vi "Temperature measurement system - main.vi"() -> ()   [LabVIEW 2022 SP3]
panel:
  in  "Speed":u32=100
  out "Thermometer":dbl(slide) caption="Temperature" scale=0.0..100.0
  out "Tea Ready":bool
  out "Elapsed Time Clock":dbl(knob) caption="Elapsed Time" scale=0.0..28800.0 scale format="%<%H:%M>t"
  out "Elapsed Time (s)":dbl format="%#_3g"
  in  "Device name":tag="myDAQ1"
  in  "B":dbl=3950.0
  in  "R0":dbl=10000.0
  in  "Stop":bool
  in  "Tab Control":enum32{"Voltage", "Resistance", "Temperature"}(tab)
  out "Voltage Chart":dbl(graph)
  out "Resistance Chart":dbl(graph)
  out "Temperature Chart":dbl(graph)
  out "Temperature":dbl format="%#_3g"
  in  "R2":dbl=10000.0
  out "Resistance":dbl
  out "Voltage 1":dbl format="%#_2g"
  out "Voltage 2":dbl format="%#_2g"
  # "Configuration"
  # "Results"
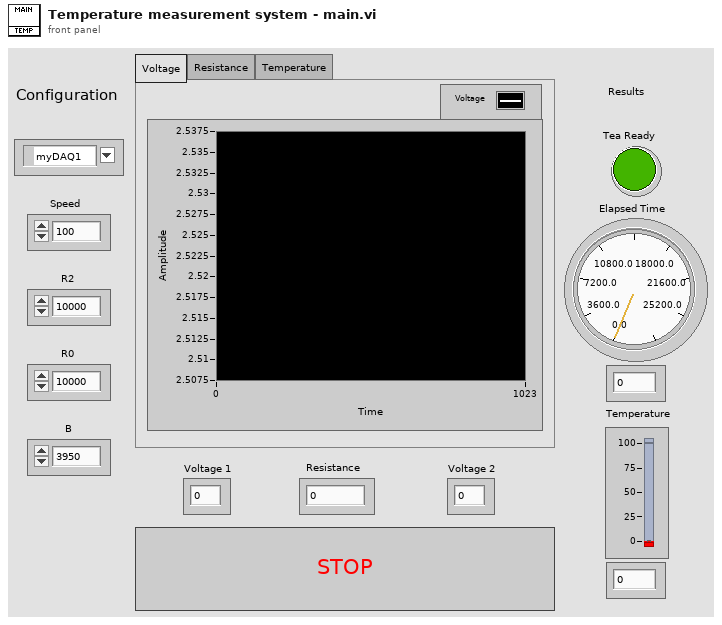
[diagram p1: front panel]
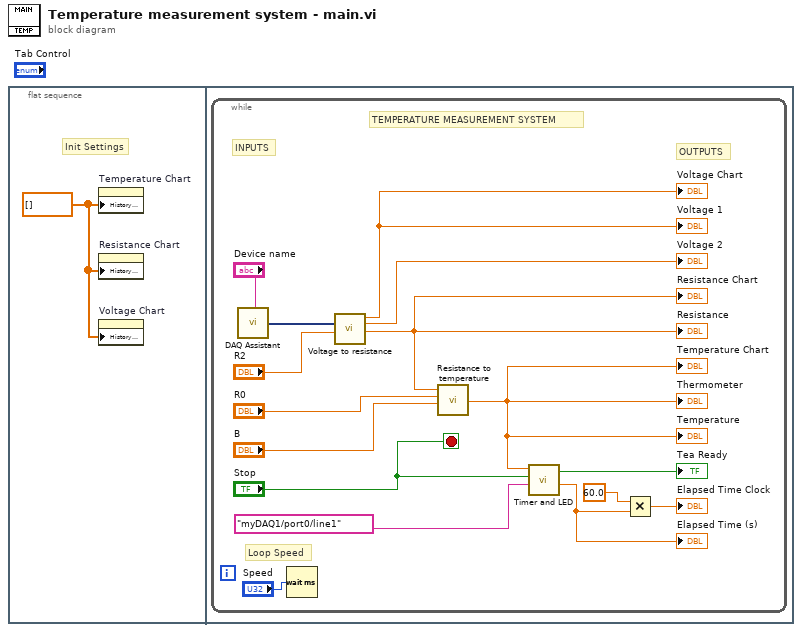
[diagram p0: block diagram]
diagram:
  n1 = flat-sequence {
    frame #0 {
      w1 = dbl[] [] ("History Data")
      # "Init Settings"
      n2 = property on="Temperature Chart" class="WFChart (strict)"("History Data"=w1) -> ()  [unwired: 2 in, 2 out]
      n3 = property on="Resistance Chart" class="WFChart (strict)"("History Data"=w1) -> ()  [unwired: 2 in, 2 out]
      n4 = property on="Voltage Chart" class="WFChart (strict)"("History Data"=w1) -> ()  [unwired: 2 in, 2 out]
    }
    frame #1 {
      n5 = while {
        stop <- "Stop" stop-if-true
        # "TEMPERATURE MEASUREMENT SYSTEM"
        # "OUTPUTS"
        # "INPUTS"
        # "Loop Speed"
        n6 = call "DAQ Assistant"("device name"="Device name") -> ("data"=w9:dynamicdata)  [unwired: 16 in, 2 out]
        n7 = Wait (ms)(milliseconds to wait="Speed") -> ()  [unwired: 1 out]
        n8 = call "Voltage to resistance.vi"("data"=w9, "R2"="R2") -> ("Voltage 2"=→"Voltage 2":dbl, "Numeric"=w14:dbl, "Voltage 1"=→"Voltage 1" →"Voltage Chart":dbl)  [unwired: 7 in]
        "Resistance" <- w14
        "Resistance Chart" <- w14
        n9 = call "Resistance to temperature.vi"("B"="B", "Resistance"=w14, "R0"="R0") -> ("Temperature"=w8:dbl)  [unwired: 8 in]
        "Temperature" <- w8
        "Temperature Chart" <- w8
        "Thermometer" <- w8
        n10 = call "Timer and LED.vi"("lines"=tag "myDAQ1/port0/line1", "Stop"="Stop", "Temperature"=w8) -> ("Tea Ready"=→"Tea Ready":bool, "Elapsed Time (s)"=w6:dbl)  [unwired: 7 in]
        "Elapsed Time (s)" <- w6
        n11 = Multiply(x=60.0, y=w6) -> (x*y=→"Elapsed Time Clock":dbl)
      }
    }
  }
